vi "SetParam.vi"(8 "error in (no error)":errorcluster caption="entrée d'erreur (pas d'erreur)", 10 "quantile_transform":T1={"axis"=0, "n_quantiles"=1000, "output_distribution"="uniform", "ignore_implicit_zeros"=FALSE, "subsample"=100000.0, "random_state"=-1, "copy"=TRUE} {"random_state" min=-1}, 11 "quantile_transform.lvclass":refnum<class "quantile_transform.lvclass">) -> (0 "error out":errorcluster caption="sortie d'erreur", 3 "quantile_transform.lvclass":refnum<class "quantile_transform.lvclass">)   [LabVIEW 2020, in "quantile_transform.lvclass"]
doc: "Set Parameters"
uses:
  quantile_transform.lvclass
  quantile_transform.lvclass/quantile_transform.ctl
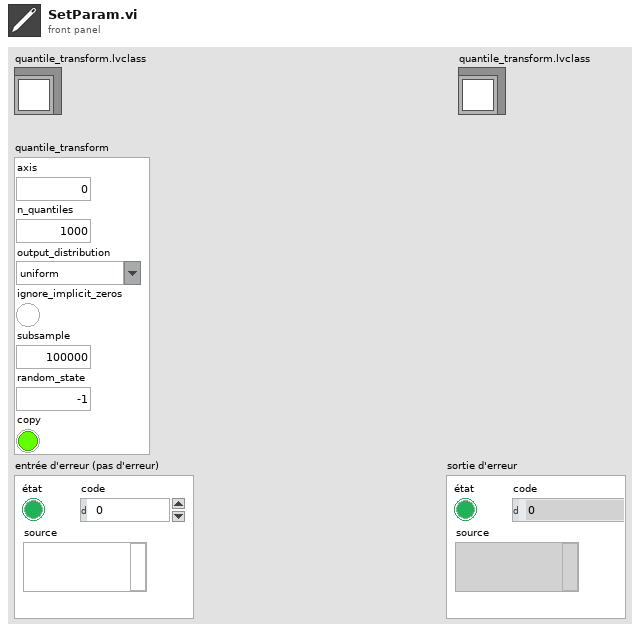
[diagram p1: front panel]
types:
  T1 = cluster{"axis":i32, "n_quantiles":i32, "output_distribution":string, "ignore_implicit_zeros":bool, "subsample":dbl, "random_state":i32, "copy":bool}
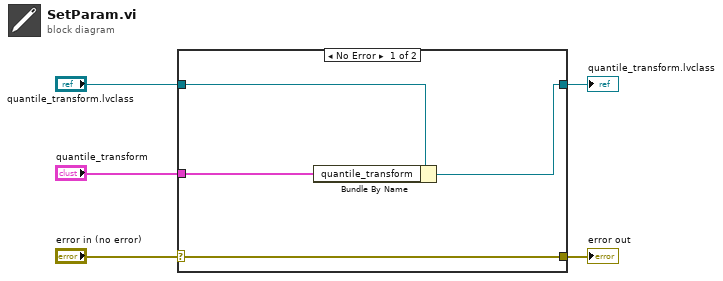
[diagram p0: block diagram]
diagram:
  n1 = case shown="No Error" "error in (no error)" {
    selector: "error in (no error)" -> [w9 w10]
    tunnel: [w9 w10] -> w4
    tunnel: [w7 w11] -> w2
    tunnel: "quantile_transform.lvclass" -> [w8 w11]
    tunnel: "quantile_transform" -> [w6 _]
    frame No Error {
      n2 = Bundle By Name(cluster=w8, "quantile_transform"=w6) -> (w7:refnum<class "quantile_transform.lvclass">)
    }
    frame Error {
    }
  }
  "error out" <- w4
  "quantile_transform.lvclass" <- w2
